vi "modify channel test.vi"() -> ()   [LabVIEW 2013, in "scan engine tests.lvlib"]
uses:
  scan engine tests.lvlib
  <vilib>/NI/Tag Bus Module Framework/channel/TBM channel.lvclass/TBM channel.ctl
  <vilib>/NI/Tag Bus Module Framework/channel/channel classification.ctl
  configuration/Scan Engine configuration.lvclass
  <vilib>/NI/Tag Bus/tag/tag descriptor.lvclass/tag descriptor.ctl
  <vilib>/NI/Tag Bus Module Framework/channel/Read channel classification.vi
  <vilib>/NI/Tag Bus Module Framework/channel/Write channel classification.vi
  <vilib>/NI/Tag Bus/tag/read tag name.vi
  <vilib>/NI/Tag Bus Module Framework/channel/TBM channel.lvclass
panel:
  out "set success":bool
  out "no err":errorcluster
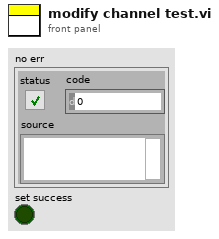
[diagram p1: front panel]
types:
  T1 = typedef "TBM channel.lvclass/channel classification.ctl" = enum16{"input data", "output data", "processing parameter", "processing result"}
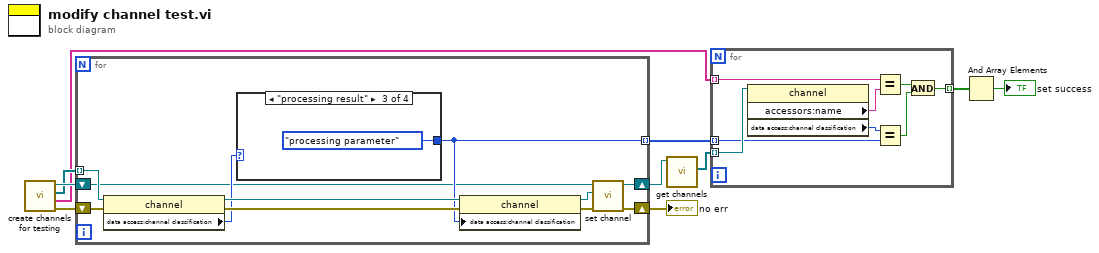
[diagram p0: block diagram]
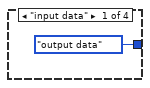
[diagram p2: hidden frame]
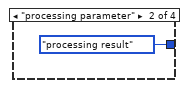
[diagram p3: hidden frame]
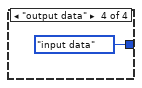
[diagram p4: hidden frame]
diagram:
  n1 = call "create channels for testing.vi"() -> ("error out"=w2:errorcluster, "names"=w1:string[], "chans"=w3:refnum<class "TBM channel.lvclass">[], "Scan Engine configuration out"=w4:refnum<class "Scan Engine configuration.lvclass">)  [unwired: 7 in, 1 out]
  n2 = for {
    shift-right: [w11] -> w10
    shift-left: w4 -> [w15]
    shift-right: [w12] -> w9
    shift-left: w2 -> [w21]
    tunnel: w3 -> [w19] mode=indexing
    tunnel: [w16] -> w5 mode=indexing
    n3 = property class="channel"(reference=w19, error in=w21) -> (reference out=w18:refnum<class "TBM channel.lvclass">, error out=w20:errorcluster, "data access:channel classification"=w17:T1)
    n4 = case shown="\"processing result\"" w17 {
      tunnel: [channel_classification."output data" ("channel classification") channel_classification."processing result" ("channel classification") channel_classification."processing parameter" ("channel classification") channel_classification."input data" ("channel classification")] -> w16
      frame "input data" {
      }
      frame "processing parameter" {
      }
      frame "processing result" {
      }
      frame "output data" {
      }
    }
    n5 = property class="channel"(reference=w18, error in=w20, "data access:channel classification"=w16) -> (reference out=w14:refnum<class "TBM channel.lvclass">, error out=w13:errorcluster)
    n6 = call "set channel.vi"("error in"=w13, "channel"=w14, "Scan Engine configuration in"=w15) -> ("error out"=w12:errorcluster, "Scan Engine configuration out"=w11:refnum<class "Scan Engine configuration.lvclass">)  [unwired: 7 in]
  }
  "no err" <- w9
  n7 = call-dynamic "get channels.vi"("module configuration in"=w10) -> ("channels"=w8:refnum<class "TBM channel.lvclass">[])  [unwired: 9 in, 1 out]
  n8 = for {
    tunnel: w8 -> [w32] mode=indexing
    tunnel: [w31] -> w7 mode=indexing
    tunnel: w5 -> [w30] mode=indexing
    tunnel: w1 -> [w27] mode=indexing
    n9 = property class="channel"(reference=w32) -> ("accessors:name"=w28:string, "data access:channel classification"=w29:T1)  [unwired: 1 in, 2 out]
    n10 = Equal?(x=w27, y=w28) -> (x = y?=w26:bool)
    n11 = Equal?(x=w29, y=w30) -> (x = y?=w33:bool)
    n12 = And(x=w26, y=w33) -> (x .and. y?=w31:bool)
  }
  n13 = And Array Elements(Boolean array=w7) -> (logical AND=→"set success":bool)
